vi "Semaphore Init.vi"(8 "error in (no error)":errorcluster, 9 "initial value (0)":u32, 10 "process (private)":T1, 11 "Semaphore in":T2) -> (0 "error out":errorcluster, 3 "Semaphore out":T2)   [LabVIEW 2013, in "POSIX Threads.lvlib" / "Semaphore.lvclass"]
doc: "Calls sem_init() on the semaphore object encapsulated by Semaphore.\n\nThis VI initializes the semaphore object and sets its default values.\n\nRefer to online POSIX documentation for more information."
uses:
  Semaphore.lvclass
  Controls/reference.ctl
  Controls/Public/C Enums/pthread_process_shared.ctl
  POSIX Thread Object/POSIX Thread Object.lvclass/POSIX Thread Object.ctl
  POSIX Thread Object/Private VIs/libpthread path.vi
  POSIX Thread Object/Private VIs/get pthread error.vi
  <vilib>/NI/NI Linux RT Errno/VIs/Public/SubVIs/errno enum to number.vi
  <vilib>/NI/NI Linux RT Errno/VIs/Public/Get Errno Value for Calling Thread.vi
  POSIX Thread Object/POSIX Thread Object.lvclass
  POSIX Threads.lvlib
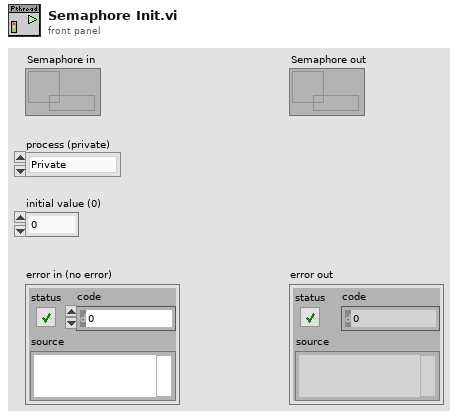
[diagram p1: front panel]
types:
  T1 = typedef "POSIX Threads.lvlib/pthread_process_shared.ctl" = enum16{"Private", "Shared"}
  T2 = typedef "POSIX Threads.lvlib/Semaphore.lvclass/reference.ctl" = refnum<data-value>
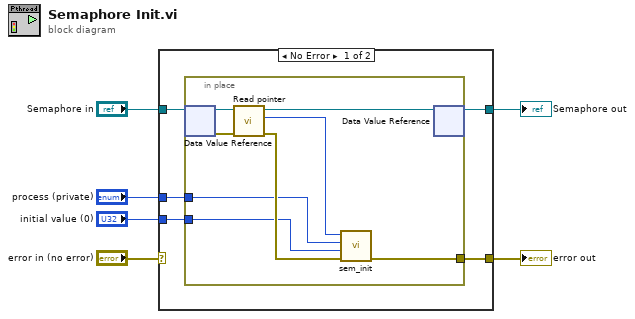
[diagram p0: block diagram]
diagram:
  n1 = case shown="No Error" "error in (no error)" {
    selector: "error in (no error)" -> [_ w20]
    tunnel: "Semaphore in" -> [w11 w21]
    tunnel: [w10 w21] -> w3
    tunnel: [w9 w20] -> w4
    tunnel: "process (private)" -> [w7 _]
    tunnel: "initial value (0)" -> [w8 _]
    frame No Error {
      n2 = in-place {
        in-place-border: [w16] -> w9
        in-place-border: w8 -> [w13]
        in-place-border: w7 -> [w12]
        n3 = in-place-dvr #1(w11) -> (w19:refnum<class "Semaphore.lvclass">, w18:errorcluster)
        n4 = call "Read pointer.vi"("error in (no error)"=w18, "POSIX Thread Object in"=w19) -> ("error out"=w15:errorcluster, "pointer"=w14:u64, "POSIX Thread Object out"=w17:refnum<class "Semaphore.lvclass">)  [unwired: 7 in]
        n5 = call "sem_init.vi"("error in (no error)"=w15, "initial value (0)"=w13, "process (private)"=w12, "sempahore ptr in"=w14) -> ("error out"=w16:errorcluster)  [unwired: 6 in, 1 out]
        n6 = in-place-dvr #1(w17) -> (w10:T2)  [unwired: 1 out]
      }
    }
    frame Error {
    }
  }
  "error out" <- w4
  "Semaphore out" <- w3
